vi "save_fp_openg.vi"(8 "error in (no error)":errorcluster, 11 "VI in":refnum<vi>) -> (0 "error out":errorcluster)   [LabVIEW 2018]
uses:
  <vilib>/Utility/config.llb/NI_LVConfig.lvlib
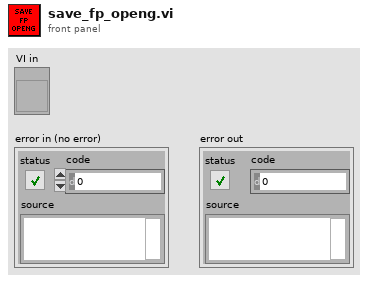
[diagram p1: front panel]
types:
  T1 = typedef "NI_LVConfig.lvlib/Config Data RefNum.ctl" = refnum<k1>
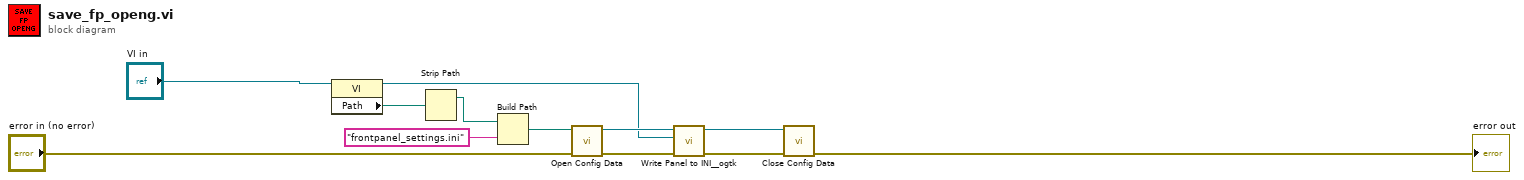
[diagram p0: block diagram]
diagram:
  n1 = property class="VI"(reference="VI in") -> (reference out=w5:refnum<vi>, "Path"=w1:path)  [unwired: 1 in, 1 out]
  n2 = Strip Path(path=w1) -> (stripped path=w3:path)  [unwired: 1 out]
  n3 = Build Path(base path=w3, name or relative path="frontpanel_settings.ini") -> (appended path=w7:path)
  n4 = call <vilib>:"Open Config Data.vi"("error in (no error)"="error in (no error)", "configuration file path"=w7) -> ("error out"=w9:errorcluster, "refnum"=w6:T1)  [unwired: 7 in, 1 out]
  n5 = call <userlib>:"Write Panel to INI__ogtk.vi"("error in (no error)"=w9, "VI ref"=w5, "refnum"=w6) -> ("error out"=w10:errorcluster, "refnum out"=w12:T1)  [unwired: 7 in]
  n6 = call <vilib>:"Close Config Data.vi"("error in (no error)"=w10, "refnum"=w12) -> ("error out"=→"error out":errorcluster)  [unwired: 8 in, 1 out]
